vi "PD500 - E-Stop.vi"(8 "error in (no error)":errorcluster, 10 "Message IN":string) -> (0 "error out":errorcluster, 1 "Result (bool)":bool, 2 "Message OUT":string, 3 "VISA OUT":refnum<visa-resource-name>)   [LabVIEW 2022 SP3]
uses:
  <vilib>/DAQmx/write.llb/DAQmx Write (Digital Bool 1Line 1Point).vi
  <vilib>/DAQmx/miscellaneous.llb/DAQmx Fill In Error Info.vi
panel:
  out "Result (color)":u32(colorbox)
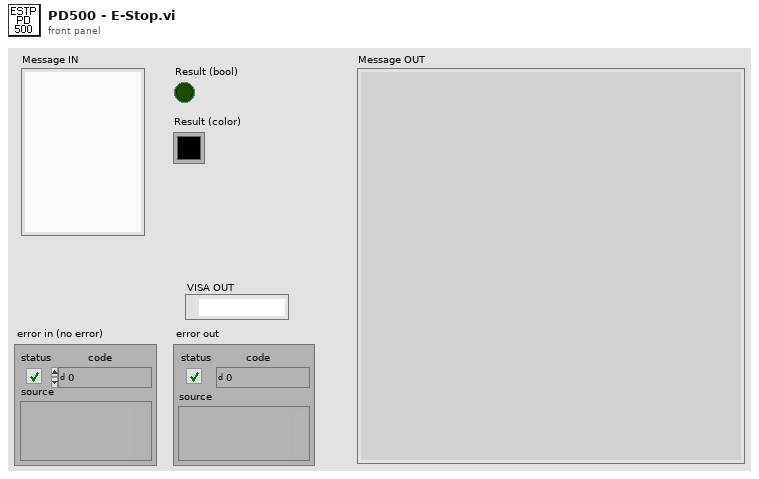
[diagram p1: front panel]
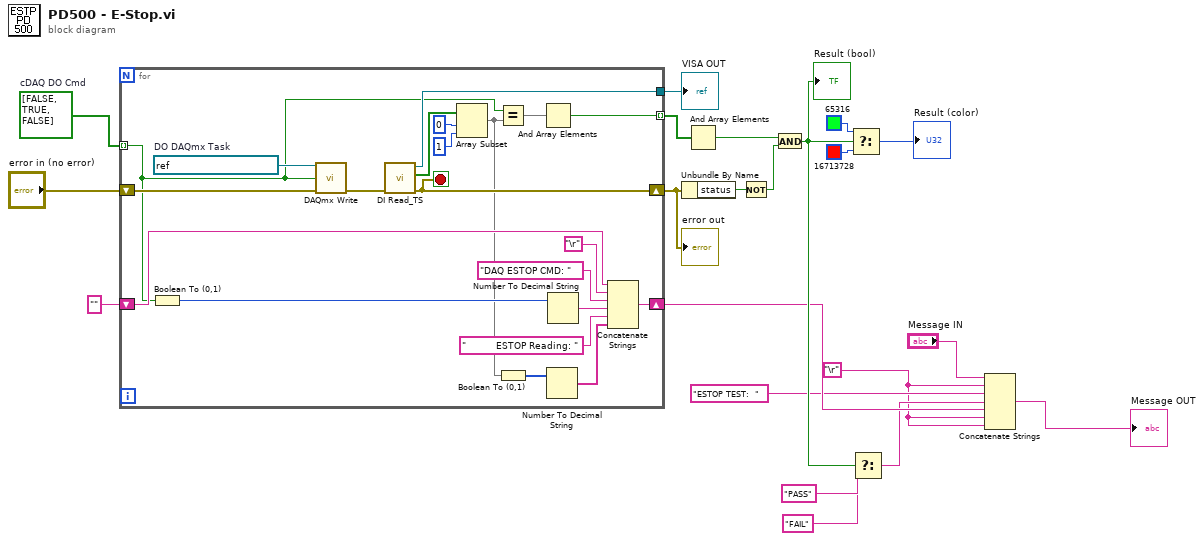
[diagram p0: block diagram]
diagram:
  w1 = bool[] [FALSE, TRUE, FALSE]  # cDAQ DO Cmd
  w3 = "\r"
  n1 = for {
    shift-right: [w37] -> w13
    shift-left: "error in (no error)" -> [w42]
    tunnel: [w41] -> w15
    tunnel: [w40] -> w14 mode=indexing
    shift-right: [w29] -> w8
    shift-left: "" -> [w28]
    tunnel: w1 -> [w22] mode=indexing
    stop <- w37 stop-if-true
    w38 = refnum<k21> "FTS2_PD500_EStop"  # DO DAQmx Task
    n2 = Boolean To (0,1)(Boolean=w22) -> (0, 1=w31:i16)
    n3 = call-poly <vilib>:"DAQmx Write.vi"("task/channels in"=w38, "data"=w22, "error in"=w42) -> ("error out"=w27:errorcluster)  [unwired: 10 in, 2 out]
    n4 = call "DI Read_TS.vi"("error in (no error)"=w27) -> ("error out"=w37:errorcluster, "DI Reading"=w24:bool[], "VISA Refnum out"=w41:refnum<visa-resource-name>)  [unwired: 7 in, 1 out]
    n5 = Array Subset(array=w24, index=0, length=1) -> (w23:bool[])
    n6 = Equal?(x=w22, y=w23) -> (x = y?=w39:bool[])
    n7 = Boolean To (0,1)(Boolean=w23) -> (0, 1=w30:i16[])
    n8 = And Array Elements(Boolean array=w39) -> (logical AND=w40:bool)
    n9 = Number To Decimal String(number=w30) -> (decimal integer string=w36:string[])  [unwired: 1 in]
    n10 = Number To Decimal String(number=w31) -> (decimal integer string=w34:string)  [unwired: 1 in]
    n11 = Concatenate Strings(w28, "\r", "DAQ ESTOP CMD: ", w34, "          ESTOP Reading: ", w36) -> (w29:string)
  }
  "error out" <- w13
  "VISA OUT" <- w15
  n12 = Unbundle By Name(w13) -> ("status"=w12:bool)
  n13 = And Array Elements(Boolean array=w14) -> (logical AND=w10:bool)
  n14 = Not(x=w12) -> (.not. x?=w9:bool)
  n15 = And(x=w10, y=w9) -> (x .and. y?=w11:bool)
  "Result (bool)" <- w11
  n16 = Select(t=u32 65316 ("Result (color)"), s=w11, f=u32 16713728 ("Result (color)")) -> (s? t:f=→"Result (color)":u32)
  n17 = Select(t="PASS", s=w11, f="FAIL") -> (s? t:f=w5:string)
  n18 = Concatenate Strings("Message IN", w3, "ESTOP TEST:  ", w5, w8, w3, w3) -> (→"Message OUT":string)
